vi "ValveGlobals.vi"() -> ()   [LabVIEW 2016]
panel:
  out "Volume Remaining":dbl[](array[numeric])
  out "Pressure Changes (mbar)":dbl[](array[numeric])
  in  "Total Odor Flow":dbl=425.0
  in  "Total Flow Setpoint":dbl=531.25
  in  "Ctr Water Valve":u16(ring)=15 items=["A1", "A2", "A3", "A4", "B1", "B2", "B3", "B4", "B5", "B6", "B7", "B8", "A5", "A6", "A7", "A8"]
  in  "Ctr Odor Valve":u16(ring)=14 items=["A1", "A2", "A3", "A4", "B1", "B2", "B3", "B4", "B5", "B6", "B7", "B8", "A5", "A6", "A7", "A8"]
  out "Pressure Group":u8[](array[numeric])=[3, 3, 3, 3, 4, 4, 4, 4]
  in  "Valves Used":u16[](array[ring])=[0, 1, 2, 3, 8, 9, 10, 11] items=["A1", "A2", "A3", "A4", "B1", "B2", "B3", "B4", "B5", "B6", "B7", "B8"]
  in  "Valves":bool[][](array[boolean])=[[FALSE, FALSE, FALSE], [FALSE, FALSE, FALSE], [FALSE, FALSE, FALSE], [FALSE, FALSE, FALSE], [FALSE, FALSE, FALSE], [FALSE, FALSE, FALSE], [FALSE, FALSE, FALSE], [FALSE, FALSE, FALSE]]
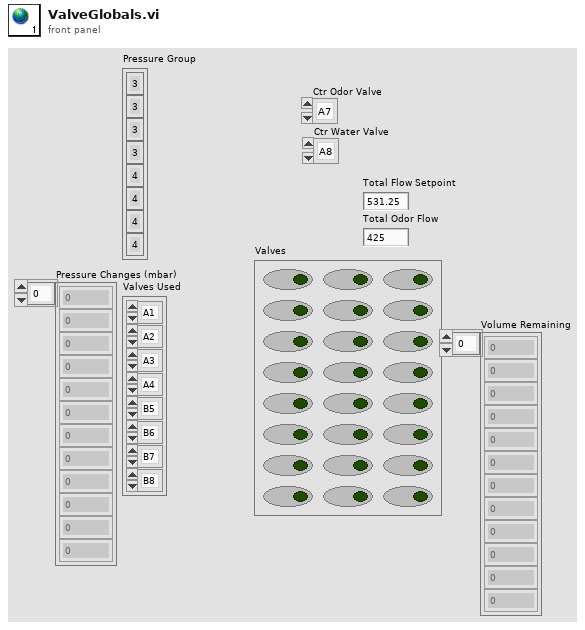
[diagram p1: front panel]
diagram:
